vi "WriteToFile.vi"(8 "error in (no error)":errorcluster, 10 "File Name":path, 11 "Workbook Reference":refnum<k24>) -> (0 "error out":errorcluster, 3 "Workbook Reference Out":refnum<k24>)   [LabVIEW 2013]
uses:
  C:/PhaeronGit/LVNPOI/Resources/NPOI 2.1.1 dotnet2/NPOI.dll
  Resources/NPOI 2.1.1 dotnet2/NPOI.dll
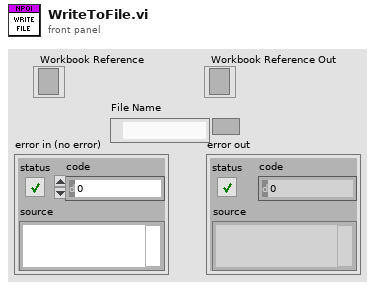
[diagram p1: front panel]
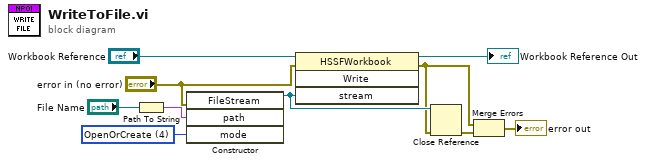
[diagram p0: block diagram]
diagram:
  w8 = 4 items=["CreateNew"=1, "Create"=2, "Open"=3, "OpenOrCreate"=4, "Truncate"=5, "Append"=6] ("mode")
  n1 = Path To String(path="File Name") -> (string=w9:string)
  n2 = constructor class="FileStream"(error in="error in (no error)", "path"=w9, "mode"=w8) -> (reference out=w4:refnum<k24>)  [unwired: 2 in, 4 out]
  n3 = invoke class="HSSFWorkbook" method="Write"(reference="Workbook Reference", error in="error in (no error)", "stream"=w4) -> (reference out=→"Workbook Reference Out":refnum<k24>, error out=w3:errorcluster)  [unwired: 1 in, 2 out]
  n4 = Close Reference(reference=w4, error in (no error)=w3) -> (error out=w1:errorcluster)
  n5 = Merge Errors(w3, w1) -> (→"error out":errorcluster)
